vi "HAPS_LoadTable_Manual_Selected_Any_Preamp_Gain.vi"() -> ()   [LabVIEW 2023, in "HAPS.lvlib"]
uses:
  HAPS.lvlib
  set_ele.ctl
  HAPS_SerialPort.ctl
  HAPS_MCU_ELE_Func.ctl
  <vilib>/Utility/file.llb/Read Delimited Spreadsheet (string).vi
  R_S/R_S.lvlib
panel:
  in  "Load Gain?":bool
  in  "file path":path=path "D:/_Project/_Code/LabVIEW/_CLC_Gen4/CLC_LV2023/CLC_Cali/Log/HAPS/Preset.csv"
  in  "Preamp_Channel":bool[](array[boolean])
  in  "offset":i32=16
  in  "H_V?":bool
  in  "IC_On/OFF":bool[][](array[boolean])=[[FALSE, FALSE, FALSE, FALSE, FALSE, FALSE, FALSE, FALSE, FALSE, FALSE, FALSE, FALSE], [FALSE, FALSE, FALSE, FALSE, FALSE, FALSE, FALSE, FALSE, FALSE, FALSE, FALSE, FALSE], [FALSE, FALSE, FALSE, FALSE, FALSE, FALSE, FALSE, FALSE, FALSE, FALSE, FALSE, FALSE]]
  in  "ele_gain?":i32=35
  in  "sys reboot?":bool=TRUE
  in  "VISA resource name":refnum<visa-resource-name>="COM1"
  out "error IO":errorcluster
  out "Err_code":i32
  out "status":bool
  in  "offset?":bool
  in  "simu.?":bool
  in  "set_ele":T1={"ch"=0, "chain_id"=0, "group"=0, "array_id"=0, "ele_phase"=0, "ele_gain"=35, "com_gain"=17, "pd_range"=0}
  out "ele phase":i32
  out "ele gain":i32
  out "channel":i32
  out "chain ID":i32
  out "group":i32
  out "array id":i32
  # "HAPS 24x24 Setting Manual In-Phase : \n                               Any BFIC & Preamp & Gain"
  # "Tx:35\nRx:22"
  # "0"
  # "5"
  # "6"
  # "11"
  # "Group_0"
  # "Group_1"
  # "Group_2"
  # "Not using!!!!!!!!!!!!!!!!!!!!!!!!!!!!!!!!!!!!!!!!"
  # "0        1       2        3        4       5        6       7        8        9      10      11     12     13     14      15"
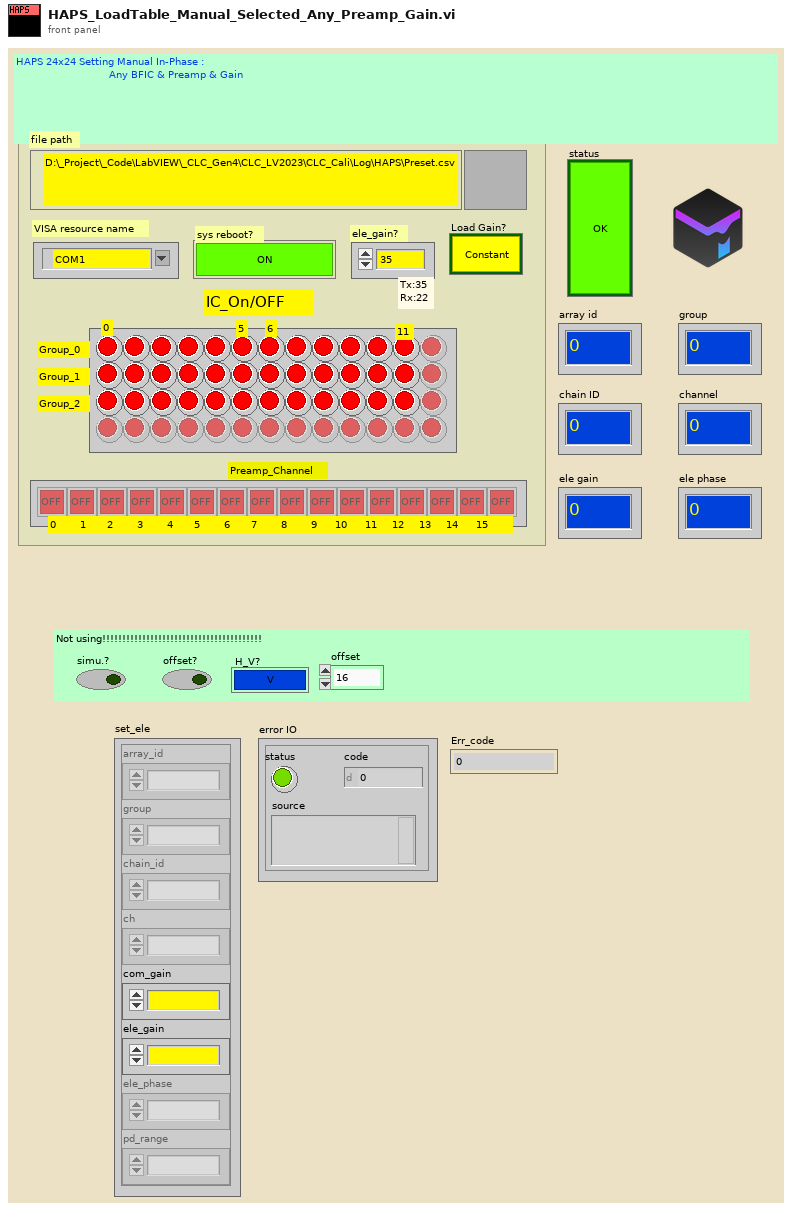
[diagram p1: front panel]
types:
  T1 = typedef "HAPS.lvlib/set_ele.ctl" = cluster{"ch":i32, "chain_id":i32, "group":i32, "array_id":i32, "ele_phase":i32, "ele_gain":i32, "com_gain":i32, "pd_range":i32}
  T2 = typedef "HAPS.lvlib/HAPS_SerialPort.ctl" = enum16{"Init", "Close", "CMD", "Flush"}
  T3 = typedef "HAPS.lvlib/HAPS_MCU_ELE_Func.ctl" = enum16{"array_init", "set_com_gain", "set_ch_gain_phase", "set_pd_range", "get_preamp_temp", "get_bfic_temp", "get_tx_pd", "ch_on", "ch_on_2", "ch_ctrl_all", "array_ctrl_src"}
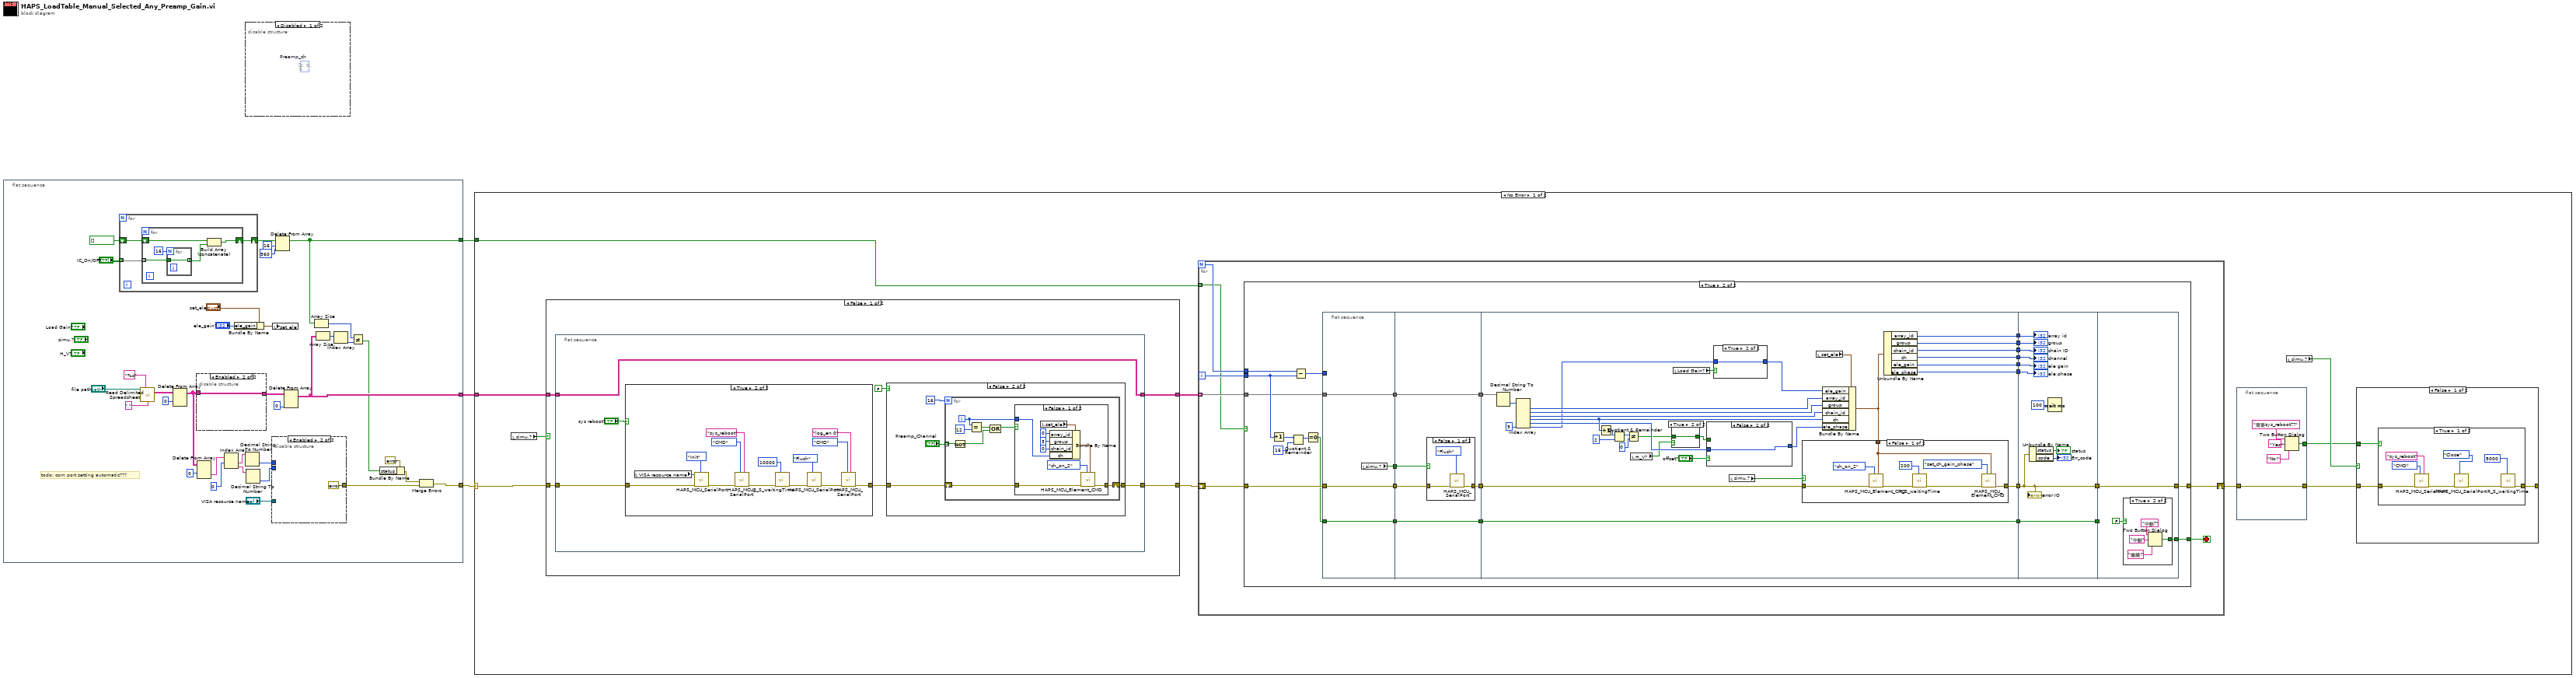
[diagram p0: block diagram]
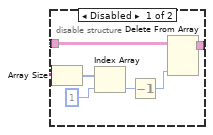
[diagram p2: hidden frame]
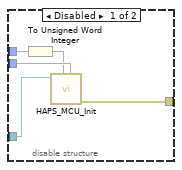
[diagram p3: hidden frame]
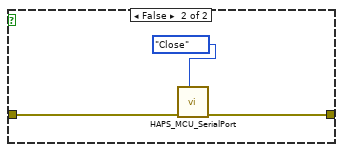
[diagram p5: hidden frame]
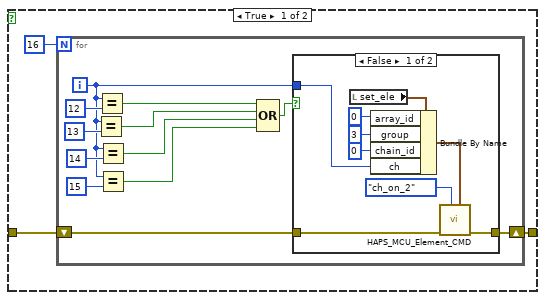
[diagram p7: hidden frame]
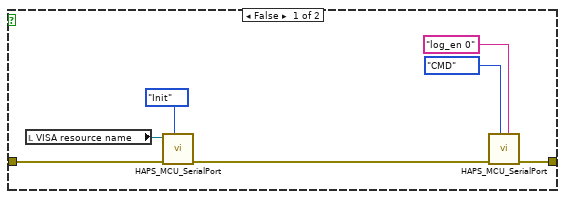
[diagram p10: hidden frame]
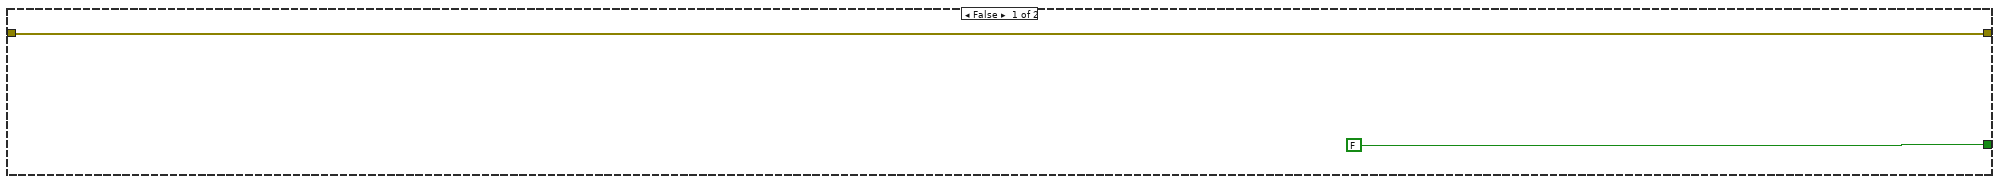
[diagram p12: hidden frame]
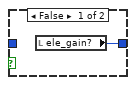
[diagram p14: hidden frame]
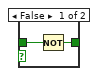
[diagram p15: hidden frame]
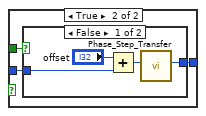
[diagram p16: hidden frame]
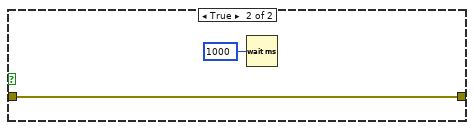
[diagram p18: hidden frame]
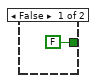
[diagram p19: hidden frame]
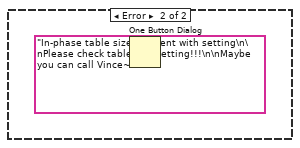
[diagram p20: hidden frame]
diagram:
  n1 = flat-sequence {
    tunnel: [w7] -> w3
    tunnel: [w11] -> w2
    tunnel: [w12] -> w1
    frame #0 {
      # "todo: com port setting automatic???"
      n2 = for {
        tunnel: "IC_On/OFF" -> [w47] mode=indexing
        shift-right: [w45] -> w17
        shift-left: bool[] [] -> [w46]
        n3 = for {
          tunnel: w47 -> [w51] mode=indexing
          shift-right: [w48] -> w45
          shift-left: w46 -> [w49]
          n4 = for {
            N: 16 -> [_]
            tunnel: w51 -> [w53]
            tunnel: [w53] -> w50 mode=indexing
          }
          n5 = Build Array (concatenate)(w49, w50) -> (w48:bool[])
        }
      }
      n6 = call-poly <vilib>:"Read Delimited Spreadsheet.vi"("file path (dialog if empty)"="file path", "format (%s)"="%s" ("format (%.3f)"), "delimiter (\\t)"="," ("delimiter (\\t)")) -> ("all rows"=w35:string[][])  [unwired: 7 in, 5 out]
      n7 = Delete From Array(array=w35, index (row)=0) -> (array with subset deleted=w29:string[][])  [unwired: 2 in, 1 out]
      n8 = disable-structure shown="Enabled" {
        disable-tunnel: [w39 w44] -> w32
        disable-tunnel: w29 -> [w38 w44]
        frame Disabled {
          n9 = Array Size(array=w38) -> (size(s)=w43:i32[])
          n10 = Index Array(array=w43, index=1) -> (element=w40:i32)
          n11 = Decrement(x=w40) -> (x-1=w42:i32)
          n12 = Delete From Array(array=w38, index (col)=w42) -> (array with subset deleted=w39:string[][])  [unwired: 2 in, 1 out]
        }
        frame Enabled {
        }
      }
      n13 = Delete From Array(array=w29, index (row)=0) -> (deleted portion=w28:string[])  [unwired: 2 in, 1 out]
      n14 = Index Array(array=w28, index #1=0 ("index")) -> (element #1=w27:string, element #2=w26:string)  [unwired: 1 in]
      n15 = Bundle By Name(cluster="set_ele", "ele_gain"="ele_gain?") -> (w18:T1)
      n16 = Decimal String To Number(string=w27) -> (number=w23:i32)  [unwired: 2 in, 1 out]
      n17 = Decimal String To Number(string=w26) -> (number=w22:i32)  [unwired: 2 in, 1 out]
      n18 = disable-structure shown="Enabled" {
        disable-tunnel: [w58 errorcluster {"status"=FALSE, "code"=0, "source"=""} ("error out")] -> w33
        disable-tunnel: w23 -> [w57 _]
        disable-tunnel: w22 -> [w56 _]
        disable-tunnel: "VISA resource name" -> [w55 _]
        frame Disabled {
          n19 = To Unsigned Word Integer(number=w57) -> (unsigned 16bit integer=w54:u16)
          n20 = call "HAPS_MCU_Init.vi"("array_id"=w56, "Tx/Rx"=w54, "VISA resource name"=w55) -> ("error out"=w58:errorcluster)  [unwired: 8 in]
        }
        frame Enabled {
        }
      }
      n21 = local write "set_ele"(w18) -> ()
      n22 = Delete From Array(array=w17, length=16, index=560) -> (array with subset deleted=w12:bool[])  [unwired: 1 out]
      n23 = Delete From Array(array=w32, index (col)=0 ("index (row)")) -> (array with subset deleted=w11:string[][])  [unwired: 2 in, 1 out]
      n24 = Array Size(array=w12) -> (size(s)=w9:i32)
      n25 = Array Size(array=w11) -> (size(s)=w10:i32[])
      n26 = Index Array(array=w10) -> (element=w8:i32)  [unwired: 1 in]
      n27 = Not Equal?(x=w9, y=w8) -> (x != y?=w5:bool)
      n28 = Bundle By Name(cluster=errorcluster {"status"=FALSE, "code"=0, "source"=""} ("error out"), "status"=w5) -> (w4:errorcluster)
      n29 = Merge Errors(w4, w33) -> (w7:errorcluster)
    }
  }
  n30 = disable-structure shown="Disabled" {
    frame Disabled {
      (unwired) i32[][] [[2, 0, 0, 8, 8, 10, 11, 9, 9, 1, 1, 3], [3, 1, 1, 9, 9, 11, 13, 15, 15, 7, 7, 5], [5, 7, 7, 15, 15, 13, 14, 14, 6, 6, 4, 12]]  # Preamp_ch
    }
    frame Enabled {
    }
  }
  n31 = case shown="No Error" w3 {
    selector: w3 -> [w67 _]
    tunnel: w2 -> [w69 _]
    tunnel: w1 -> [w63 _]
    frame No Error {
      n32 = local read "simu.?"() -> (w65:bool)
      n33 = case shown="False" w65 {
        tunnel: w69 -> [w93 w169]
        tunnel: [w92 w169] -> w68
        tunnel: w67 -> [w91 w168]
        tunnel: [w90 w168] -> w66
        frame False {
          n34 = flat-sequence {
            tunnel: w93 -> [w99]
            tunnel: [w99] -> w92
            tunnel: w91 -> [w97]
            tunnel: [w98] -> w90
            frame #0 {
              n35 = case shown="True" "sys reboot?" {
                tunnel: w97 -> [w151 w165]
                tunnel: [w149 w163] -> w96
                frame False {
                  n36 = local read "VISA resource name"() -> (w147:refnum<visa-resource-name>)
                  n37 = call "HAPS_MCU_SerialPort.vi"("HAPS_SerialPort_Func"=HAPS_SerialPort."Init", "error in"=w151, "VISA resource name"=w147) -> ("error out"=w148:errorcluster)  [unwired: 6 in, 2 out]
                  n38 = call "HAPS_MCU_SerialPort.vi"("Command"="log_en 0", "HAPS_SerialPort_Func"=enum16{"Init", "Close", "CMD"}."CMD" ("HAPS_SerialPort"), "error in"=w148) -> ("error out"=w149:errorcluster)  [unwired: 6 in, 2 out]
                }
                frame True {
                  n39 = local read "VISA resource name"() -> (w154:refnum<visa-resource-name>)
                  n40 = call "HAPS_MCU_SerialPort.vi"("HAPS_SerialPort_Func"=HAPS_SerialPort."Init", "error in"=w165, "VISA resource name"=w154) -> ("error out"=w160:errorcluster)  [unwired: 6 in, 2 out]
                  n41 = call "HAPS_MCU_SerialPort.vi"("Command"="sys_reboot", "HAPS_SerialPort_Func"=enum16{"Init", "Close", "CMD"}."CMD" ("HAPS_SerialPort"), "error in"=w160) -> ("error out"=w159:errorcluster)  [unwired: 6 in, 2 out]
                  n42 = call "R_S_waitingTime.vi"("Waiting Time(ms)"=u32 10000, "error in"=w159) -> ("error out"=w157:errorcluster)  [unwired: 9 in]
                  n43 = call "HAPS_MCU_SerialPort.vi"("HAPS_SerialPort_Func"=HAPS_SerialPort."Flush", "error in"=w157) -> ("error out"=w155:errorcluster)  [unwired: 7 in, 2 out]
                  n44 = call "HAPS_MCU_SerialPort.vi"("Command"="log_en 0", "HAPS_SerialPort_Func"=enum16{"Init", "Close", "CMD"}."CMD" ("HAPS_SerialPort"), "error in"=w155) -> ("error out"=w163:errorcluster)  [unwired: 6 in, 2 out]
                }
              }
              n45 = case shown="False" FALSE {
                tunnel: [w101 w127] -> w98
                tunnel: w96 -> [w100 w126]
                frame True {
                  n46 = for {
                    N: 16 -> [_]
                    shift-right: [w113] -> w101
                    shift-left: w100 -> [w114]
                    i -> [w104]
                    n47 = Equal?(x=w104, y=13) -> (x = y?=w108:bool)
                    n48 = Equal?(x=w104, y=12) -> (x = y?=w112:bool)
                    n49 = Equal?(x=w104, y=14) -> (x = y?=w106:bool)
                    n50 = Equal?(x=w104, y=15) -> (x = y?=w103:bool)
                    n51 = Compound Arithmetic op=OR(w112, w108, w106, w103) -> (w109:bool)
                    n52 = case shown="False" w109 {
                      tunnel: w114 -> [w117 w124]
                      tunnel: [w116 w124] -> w113
                      tunnel: w104 -> [w115 _]
                      frame False {
                        n53 = local read "set_ele"() -> (w119:T1)
                        n54 = Bundle By Name(cluster=w119, "array_id"=0, "group"=3, "chain_id"=0, "ch"=w115) -> (w120:T1)
                        n55 = call "HAPS_MCU_Element_CMD.vi"("set_ele"=w120, "HAPS_MCU_ELE_Func."=HAPS_MCU_ELE_Func."ch_on_2", "error in"=w117) -> ("error out"=w116:errorcluster)  [unwired: 7 in, 1 out]
                      }
                      frame True {
                      }
                    }
                  }
                }
                frame False {
                  n56 = for {
                    N: 16 -> [_]
                    shift-right: [w135] -> w127
                    shift-left: w126 -> [w136]
                    tunnel: "Preamp_Channel" -> [w130] mode=indexing
                    i -> [w133]
                    n57 = Not(x=w130) -> (.not. x?=w129:bool)
                    n58 = Equal?(x=w133, y=12) -> (x = y?=w132:bool)
                    n59 = Compound Arithmetic op=OR(w132, w129) -> (w131:bool)
                    n60 = case shown="False" w131 {
                      tunnel: w136 -> [w139 w146]
                      tunnel: [w138 w146] -> w135
                      tunnel: w133 -> [w137 _]
                      frame False {
                        n61 = local read "set_ele"() -> (w141:T1)
                        n62 = Bundle By Name(cluster=w141, "array_id"=0, "group"=3, "chain_id"=0, "ch"=w137) -> (w142:T1)
                        n63 = call "HAPS_MCU_Element_CMD.vi"("set_ele"=w142, "HAPS_MCU_ELE_Func."=HAPS_MCU_ELE_Func."ch_on_2", "error in"=w139) -> ("error out"=w138:errorcluster)  [unwired: 7 in, 1 out]
                      }
                      frame True {
                      }
                    }
                  }
                }
              }
            }
          }
        }
        frame True {
        }
      }
      n64 = for {
        N -> [w174]
        tunnel: w68 -> [w172] mode=indexing
        shift-right: [w176] -> w62
        shift-left: w66 -> [w175]
        tunnel: w63 -> [w170] mode=indexing
        i -> [w173]
        stop <- w171 stop-if-true
        n65 = case shown="True" w170 {
          tunnel: [w177 w190] -> w176
          tunnel: w175 -> [w177 w189]
          tunnel: w174 -> [_ w188]
          tunnel: w173 -> [_ w187]
          tunnel: w172 -> [_ w186]
          tunnel: [FALSE ("T button?") w180] -> w171
          frame False {
          }
          frame True {
            n66 = Increment(x=w187) -> (x+1=w184:i32)
            n67 = Quotient & Remainder(x=w184, y=16) -> (x-y*floor(x/y)=w182:i32)  [unwired: 1 out]
            n68 = Subtract(x=w188, y=w187) -> (x-y=w185:i32)
            n69 = Equal To 0?(x=w182) -> (x = 0?=w181:bool)
            n70 = flat-sequence {
              tunnel: w185 -> [_]
              tunnel: w189 -> [w209]
              tunnel: w186 -> [w210]
              tunnel: [w210] -> w206
              tunnel: [w209] -> w205
              tunnel: w181 -> [w208]
              tunnel: [w208] -> w204
              tunnel: [w207] -> w179
              tunnel: [w215] -> w203
              tunnel: [w214] -> w202
              tunnel: w206 -> [w215]
              tunnel: w205 -> [w213]
              tunnel: w204 -> [w212]
              tunnel: [w212] -> w201
              tunnel: w179 -> [w211]
              tunnel: w203 -> [w251]
              tunnel: w202 -> [w249]
              tunnel: [w237] -> w200
              tunnel: [w247] -> w199
              tunnel: [w246] -> w198
              tunnel: [w245] -> w197
              tunnel: [w244] -> w196
              tunnel: [w243] -> w195
              tunnel: [w242] -> w194
              tunnel: w201 -> [w238]
              tunnel: [w238] -> w193
              tunnel: w200 -> [w278]
              tunnel: w199 -> [w286]
              tunnel: w198 -> [w285]
              tunnel: w197 -> [w284]
              tunnel: w196 -> [w283]
              tunnel: w195 -> [w282]
              tunnel: w194 -> [w281]
              tunnel: [w278] -> w192
              tunnel: w193 -> [w279]
              tunnel: [w279] -> w191
              tunnel: w192 -> [w289]
              tunnel: w191 -> [_]
              tunnel: [w289] -> w190
              tunnel: [w288] -> w180
              frame #0 {
                n71 = local read "simu.?"() -> (w207:bool)
              }
              frame #1 {
                n72 = case shown="False" w211 {
                  tunnel: [w218 w219] -> w214
                  tunnel: w213 -> [w217 w219]
                  frame False {
                    n73 = call "HAPS_MCU_SerialPort.vi"("HAPS_SerialPort_Func"=HAPS_SerialPort."Flush", "error in"=w217) -> ("error out"=w218:errorcluster)  [unwired: 7 in, 2 out]
                  }
                  frame True {
                  }
                }
              }
              frame #2 {
                n74 = Decimal String To Number(string=w251) -> (number=w250:i32[])  [unwired: 2 in, 1 out]
                n75 = Index Array(array=w250, index #6=9 ("index")) -> (element #1=w248:i32, element #2=w241:i32, element #3=w240:i32, element #4=w234:i32, element #5=w230:i32, element #6=w220:i32)  [unwired: 5 in]
                n76 = Increment(x=w234) -> (x+1=w227:i32)
                n77 = Quotient & Remainder(x=w227, y=2) -> (x-y*floor(x/y)=w232:i32)  [unwired: 1 out]
                n78 = Not Equal?(x=w232, y=0) -> (x != y?=w224:bool)
                n79 = local read "H_V?"() -> (w225:bool)
                n80 = case shown="True" w225 {
                  tunnel: w224 -> [w255 w256]
                  tunnel: [w254 w256] -> w223
                  frame False {
                    n81 = Not(x=w255) -> (.not. x?=w254:bool)
                  }
                  frame True {
                  }
                }
                n82 = local read "Load Gain?"() -> (w222:bool)
                n83 = case shown="False" "offset?" {
                  tunnel: w230 -> [w257 w260]
                  tunnel: w223 -> [_ w259]
                  tunnel: [w257 w258] -> w229
                  frame False {
                  }
                  frame True {
                    n84 = case shown="False" w259 {
                      tunnel: w260 -> [w264 w265]
                      tunnel: [w261 w265] -> w258
                      frame False {
                        n85 = Add(x="offset", y=w264) -> (x+y=w262:i32)
                        n86 = call "Phase_Step_Transfer.vi"("Input_Phase_Step"=w262) -> ("Output_Phase_Step"=w261:i32)  [unwired: 10 in]
                      }
                      frame True {
                      }
                    }
                  }
                }
                n87 = case shown="True" w222 {
                  tunnel: [w252 w253] -> w226
                  tunnel: w220 -> [_ w253]
                  frame False {
                    n88 = local read "ele_gain?"() -> (w252:i32)
                  }
                  frame True {
                  }
                }
                n89 = local read "simu.?"() -> (w236:bool)
                n90 = local read "set_ele"() -> (w239:T1)
                n91 = Bundle By Name(cluster=w239, "ele_gain"=w226, "array_id"=w248, "group"=w241, "chain_id"=w240, "ch"=w234, "ele_phase"=w229) -> (w235:T1)
                n92 = case shown="False" w236 {
                  tunnel: w249 -> [w273 w275]
                  tunnel: w235 -> [w272 _]
                  tunnel: [w271 w275] -> w237
                  frame False {
                    n93 = call "HAPS_MCU_Element_CMD.vi"("set_ele"=w272, "HAPS_MCU_ELE_Func."=HAPS_MCU_ELE_Func."ch_on_2", "error in"=w273) -> ("error out"=w267:errorcluster)  [unwired: 7 in, 1 out]
                    n94 = call "R_S_waitingTime.vi"("Waiting Time(ms)"=u32 200, "error in"=w267) -> ("error out"=w266:errorcluster)  [unwired: 9 in]
                    n95 = call "HAPS_MCU_Element_CMD.vi"("set_ele"=w272, "HAPS_MCU_ELE_Func."=HAPS_MCU_ELE_Func."set_ch_gain_phase", "error in"=w266) -> ("error out"=w271:errorcluster)  [unwired: 7 in, 1 out]
                  }
                  frame True {
                    n96 = Wait (ms)(milliseconds to wait=u32 1000) -> ()  [unwired: 1 out]
                  }
                }
                n97 = Unbundle By Name(w235) -> ("array_id"=w247:i32, "group"=w246:i32, "chain_id"=w245:i32, "ch"=w244:i32, "ele_gain"=w243:i32, "ele_phase"=w242:i32)
              }
              frame #3 {
                n98 = Unbundle By Name(w278) -> ("status"=→"status":bool, "code"=→"Err_code":i32)
                n99 = Wait (ms)(milliseconds to wait=u32 100) -> ()  [unwired: 1 out]
                "group" <- w285
                "chain ID" <- w284
                "channel" <- w283
                "ele gain" <- w282
                "ele phase" <- w281
                "array id" <- w286
                "error IO" <- w278
              }
              frame #4 {
                n100 = case shown="True" FALSE {
                  tunnel: [FALSE ("T button?") w293] -> w288
                  frame False {
                  }
                  frame True {
                    n101 = Two Button Dialog(message="中斷?", 1:"繼續!" ("F button name (\"Cancel\")"), 2:"中斷" ("T button name (\"OK\")")) -> (T button?=w293:bool)
                  }
                }
              }
            }
          }
        }
      }
      n102 = flat-sequence {
        tunnel: w62 -> [w74]
        tunnel: [w74] -> w61
        tunnel: [w70] -> w60
        frame #0 {
          n103 = Two Button Dialog(message="需要sys_reboot??", 1:"No!" ("F button name (\"Cancel\")"), 2:"Yes" ("T button name (\"OK\")")) -> (T button?=w70:bool)
        }
      }
      n104 = local read "simu.?"() -> (w64:bool)
      n105 = case shown="False" w64 {
        tunnel: [w76 w89] -> _
        tunnel: w61 -> [w77 w89]
        tunnel: w60 -> [w75 _]
        frame False {
          n106 = case shown="True" w75 {
            tunnel: w77 -> [w85 w87]
            tunnel: [w78 w86] -> w76
            frame True {
              n107 = call "HAPS_MCU_SerialPort.vi"("Command"="sys_reboot", "HAPS_SerialPort_Func"=enum16{"Init", "Close", "CMD"}."CMD" ("HAPS_SerialPort"), "error in"=w85) -> ("error out"=w81:errorcluster)  [unwired: 6 in, 2 out]
              n108 = call "HAPS_MCU_SerialPort.vi"("HAPS_SerialPort_Func"=HAPS_SerialPort."Close", "error in"=w81) -> ("error out"=w79:errorcluster)  [unwired: 7 in, 2 out]
              n109 = call "R_S_waitingTime.vi"("Waiting Time(ms)"=u32 5000, "error in"=w79) -> ("error out"=w78:errorcluster)  [unwired: 9 in]
            }
            frame False {
              n110 = call "HAPS_MCU_SerialPort.vi"("HAPS_SerialPort_Func"=HAPS_SerialPort."Close", "error in"=w87) -> ("error out"=w86:errorcluster)  [unwired: 7 in, 2 out]
            }
          }
        }
        frame True {
        }
      }
    }
    frame Error {
      n111 = One Button Dialog(message="In-phase table size different with setting\n\nPlease check table and setting!!!\n\nMaybe you can call Vince~~~") -> ()  [unwired: 1 in, 1 out]
    }
  }
